vi "Destroy.vi"(8 "error in (no error)":errorcluster, 11 "ONNX Class in":refnum<class "ONNX Class.lvclass">) -> (0 "error out":errorcluster, 3 "ONNX Class out":refnum<class "ONNX Class.lvclass">)   [LabVIEW 2017, in "ONNX Class Library.lvlib" / "ONNX Class.lvclass"]
uses:
  ONNX Class.lvclass
  ONNX Class.lvclass/ONNX Class.ctl
  ONNX Class Library.lvlib
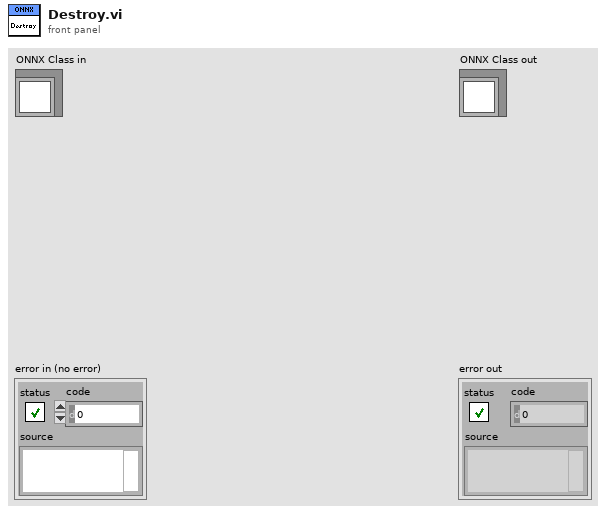
[diagram p1: front panel]
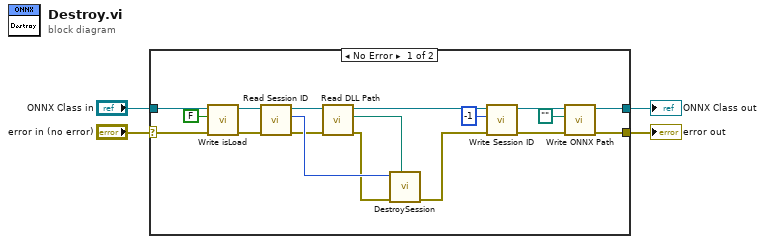
[diagram p0: block diagram]
diagram:
  n1 = case shown="No Error" "error in (no error)" {
    selector: "error in (no error)" -> [w14 w24]
    tunnel: [w7 w24] -> w3
    tunnel: [w10 w23] -> w1
    tunnel: "ONNX Class in" -> [w17 w23]
    frame No Error {
      n2 = call-dynamic "Write isLoad.vi"("error in (no error)"=w14, "isLoad"=FALSE, "ONNX Class in"=w17) -> ("error out"=w13:errorcluster, "ONNX Class out"=w16:refnum<class "ONNX Class.lvclass">)  [unwired: 7 in]
      n3 = call-dynamic "Read Session ID.vi"("error in (no error)"=w13, "ONNX Class in"=w16) -> ("error out"=w20:errorcluster, "Session ID"=w22:i32, "ONNX Class out"=w21:refnum<class "ONNX Class.lvclass">)  [unwired: 7 in]
      n4 = call-dynamic "Read DLL Path.vi"("error in (no error)"=w20, "ONNX Class in"=w21) -> ("error out"=w19:errorcluster, "DLL Path"=w18:path, "ONNX Class out"=w12:refnum<class "ONNX Class.lvclass">)  [unwired: 7 in]
      n5 = call "DestroySession.vi"("DLL path"=w18, "error in (no error)"=w19, "session id in"=w22) -> ("error out"=w9:errorcluster)  [unwired: 7 in, 1 out]
      n6 = call-dynamic "Write Session ID.vi"("error in (no error)"=w9, "Session ID"=-1, "ONNX Class in"=w12) -> ("error out"=w8:errorcluster, "ONNX Class out"=w11:refnum<class "ONNX Class.lvclass">)  [unwired: 7 in]
      n7 = call-dynamic "Write ONNX Path.vi"("error in (no error)"=w8, "ONNX Path"=path "", "ONNX Class in"=w11) -> ("error out"=w7:errorcluster, "ONNX Class out"=w10:refnum<class "ONNX Class.lvclass">)  [unwired: 7 in]
    }
    frame Error {
    }
  }
  "error out" <- w3
  "ONNX Class out" <- w1
